vi "Modbus Global.vi"(0 "HMI Coil":T1, 1 "Modbus Mode (Write Coil)":T2=enum."Write Coil", 5 "Coil IN":bool, 11 "Error IN":errorcluster) -> (4 "Coils OUT":bool[](array[boolean]), 6 "Registers OUT":u16[](array[numeric]), 15 "Error OUT":errorcluster)   [LabVIEW 2020]
uses:
  Type Defs/Modbus Mode.ctl
  Type Defs/HMI Coils.ctl
  <vilib>/NI/Modbus Library/API/Slave/Modbus Slave.lvclass
  <vilib>/NI/Modbus Library/API/Wrapper/Create Serial Slave.vi
  <vilib>/NI/Modbus Library/API/Wrapper/API Main.lvlib
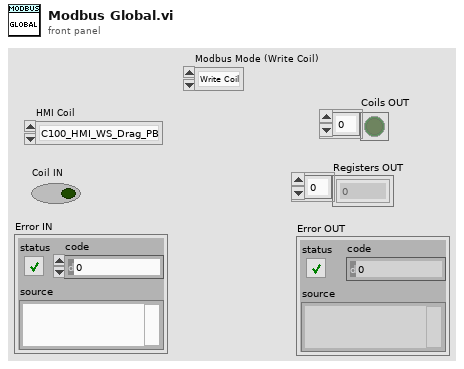
[diagram p1: front panel]
types:
  T1 = typedef "HMI Coils.ctl" = enum16{"C100_HMI_WS_Drag_PB", "C101_HMI_WB_Drag_PB", "C102_HMI_WS_Fan_PB", "C103_HMI_WB_Fan_PB", "C104_HMI_Dryr_Drag_PB", "C105_HMI_Dryr_Fan_PB", "C106_HMI_DB_Fan_PB", "C107_HMI_DB_Drag_PB", "C108_HMI_DB_Top_Feed_PB", "C109_HMI_U-Trough_PB", "C110_HMI_Leg_PB", "C111", "C112", "C113", "C114", "C115", "C116", "C117", "C118", "C119", "C220_HMI_VFD_+100_PB", "C221_HMI_VFD_+10_PB", "C222_HMI_VFD_-10_PB", "C223_HMI_VFD_-100_PB"}
  T2 = typedef "Modbus Mode.ctl" = enum16{"Init", "Read", "Write Coil", "Close"}
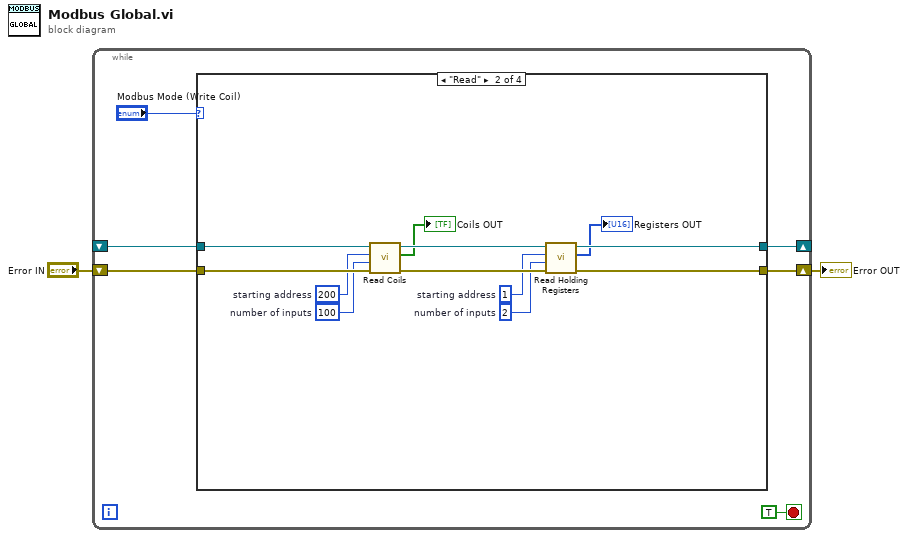
[diagram p0: block diagram]
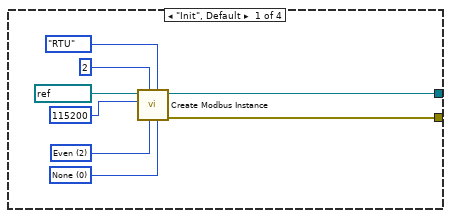
[diagram p2: hidden frame]
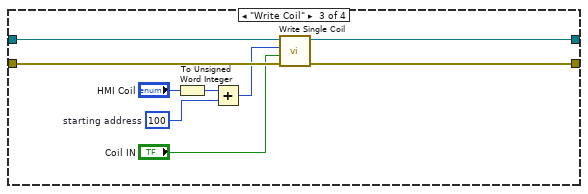
[diagram p3: hidden frame]
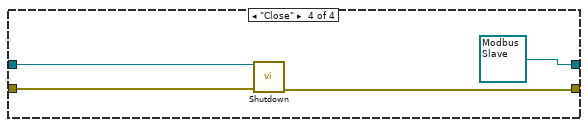
[diagram p4: hidden frame]
diagram:
  n1 = while {
    shift-right: [w6] -> _
    shift-left: _ -> [w4]
    shift-right: [w5] -> w1
    shift-left: "Error IN" -> [w3]
    stop <- TRUE stop-if-true
    n2 = case shown="\"Read\"" "Modbus Mode (Write Coil)" {
      tunnel: [w10 w24 w35 refnum<class "Modbus Slave.lvclass"> refnum ("serial slave instance")] -> w6
      tunnel: [w9 w23 w34 w39] -> w5
      tunnel: w4 -> [_ w28 w37 w41]
      tunnel: w3 -> [_ w27 w36 w40]
      frame "Init", Default {
        w16 = u16 0 items=["None", "XON/XOFF", "RTS/CTS", "XON/XOFF & RTS/CTS", "DTR/DSR", "XON/XOFF & DTR/DSR"] ("flow control")
        w14 = u16 2 items=["None", "Odd", "Even", "Mark", "Space"] ("parity (even)")
        n3 = call-poly <vilib>:"Create Modbus Instance.vi"("flow control"=w16, "serial type"=enum16{"RTU", "ASCII"}."RTU", "parity (even)"=w14, "unit ID"=u8 2, "baud rate (9600)"=u32 115200, "VISA resource name"=refnum<visa-resource-name> "COM7") -> ("error out"=w9:errorcluster, "serial slave instance"=w10:refnum<class "Modbus Slave.lvclass">)  [unwired: 4 in]
      }
      frame "Read" {
        w18 = u16 2  # number of inputs
        w19 = u16 1  # starting address
        w21 = u16 100  # number of inputs
        w22 = u16 200  # starting address
        n4 = call-dynamic "Read Coils.vi"("error in"=w27, "number of inputs"=w21, "starting address"=w22, "Modbus slave in"=w28) -> ("error out"=w25:errorcluster, "coils"=→"Coils OUT":bool[], "Modbus slave out"=w26:refnum<class "Modbus Slave.lvclass">)  [unwired: 5 in]
        n5 = call-dynamic "Read Holding Registers.vi"("error in"=w25, "number of inputs"=w18, "starting address"=w19, "Modbus slave in"=w26) -> ("error out"=w23:errorcluster, "register values"=→"Registers OUT":u16[], "Modbus slave out"=w24:refnum<class "Modbus Slave.lvclass">)  [unwired: 5 in]
      }
      frame "Write Coil" {
        w32 = u16 100  # starting address
        n6 = To Unsigned Word Integer(number="HMI Coil") -> (unsigned 16bit integer=w31:u16)
        n7 = Add(x=w31, y=w32) -> (x+y=w30:u16)
        n8 = call-dynamic "Write Single Coil.vi"("error in"=w36, "coil to write"="Coil IN", "address"=w30, "Modbus slave in"=w37) -> ("error out"=w34:errorcluster, "Modbus slave out"=w35:refnum<class "Modbus Slave.lvclass">)  [unwired: 6 in]
      }
      frame "Close" {
        n9 = call-dynamic "Shutdown.vi"("error in"=w40, "Modbus slave in"=w41) -> ("error out"=w39:errorcluster)  [unwired: 9 in]
      }
    }
  }
  "Error OUT" <- w1
